vi "STM Write Meta Data (UDP Clst).vi"(4 "Address":cluster{"address":u32, "port":u16}, 6 "Options":T3={"Ignore Timeout Error"=TRUE, "timeout ms (1000)"=1000}, 7 "Meta data":T2[](array[typedef]), 8 "error in":errorcluster, 11 "Connection Info In":T1) -> (0 "error out":errorcluster, 3 "Connection Info Out":T1)   [LabVIEW 2014, in "QwaveSys Raspberry Pi Library.lvlib"]
doc: "Use this VI to transmit the meta data cluster to a remote computer. Sending the meta data to another computer helps maintainability since the data resides only on one side and it is shared to other computers at run time."
uses:
  QwaveSys Raspberry Pi Library.lvlib
  _SubVIs/stm_MetaDataElement.ctl
  stm_UDP Connection Info.ctl
  stm_UDP Write Options.ctl
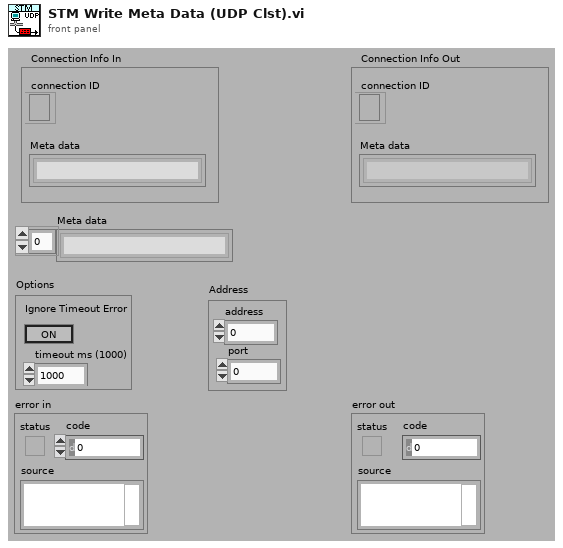
[diagram p1: front panel]
types:
  T1 = typedef "QwaveSys Raspberry Pi Library.lvlib/stm_UDP Connection Info.ctl" = cluster{"connection ID":refnum<k16>, "Meta data":T2[]}
  T2 = typedef "QwaveSys Raspberry Pi Library.lvlib/stm_MetaDataElement.ctl" = string
  T3 = typedef "QwaveSys Raspberry Pi Library.lvlib/stm_UDP Write Options.ctl" = cluster{"Ignore Timeout Error":bool, "timeout ms (1000)":i32}
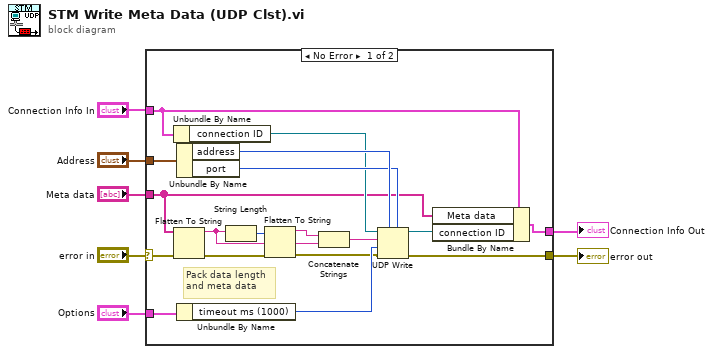
[diagram p0: block diagram]
diagram:
  n1 = case shown="No Error" "error in" {
    selector: "error in" -> [w11 w27]
    tunnel: [w12 w26] -> w7
    tunnel: "Connection Info In" -> [w14 w26]
    tunnel: "Meta data" -> [w8 _]
    tunnel: [w22 w27] -> w5
    tunnel: "Address" -> [w20 _]
    tunnel: "Options" -> [w17 _]
    frame No Error {
      # "Pack data length\nand meta data"
      n2 = Unbundle By Name(w14) -> ("connection ID"=w15:refnum<k16>)
      n3 = Flatten To String(anything=w8, error in (no error)=w11) -> (data string=w23:string, error out=w10:errorcluster)  [unwired: 3 out]
      n4 = Unbundle By Name(w20) -> ("address"=w19:u32, "port"=w18:u16)
      n5 = Unbundle By Name(w17) -> ("timeout ms (1000)"=w16:i32)
      n6 = String Length(string=w23) -> (length=w25:i32)
      n7 = Flatten To String(anything=w25, error in (no error)=w10) -> (data string=w24:string, error out=w9:errorcluster)  [unwired: 3 out]
      n8 = Concatenate Strings(w24, w23) -> (w21:string)
      n9 = UDP Write(address=w19, port or service name=w18, connection ID=w15, data in=w21, 8:w9, 9:w16) -> (error out=w22:errorcluster, 3:w13:refnum<k16>)
      n10 = Bundle By Name(cluster=w14, "Meta data"=w8, "connection ID"=w13) -> (w12:T1)
    }
    frame Error {
    }
  }
  "error out" <- w5
  "Connection Info Out" <- w7
